vi "solar_msg Q Obtain.vi"(7 "Max Queue Size (-1, unlimited)":i32=-1, 8 "error in (no error)":errorcluster, 9 "Create If Not Found? (T)":bool=TRUE, 11 "Queue Name (unnamed)":string) -> (0 "error out":errorcluster, 1 "Created New?":bool, 3 "Queue":refnum<queue>)   [LabVIEW 2018]
doc: "This obtains a queue reference by name."
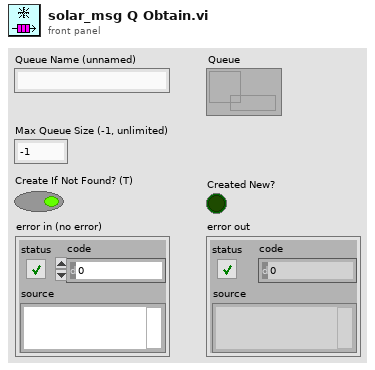
[diagram p1: front panel]
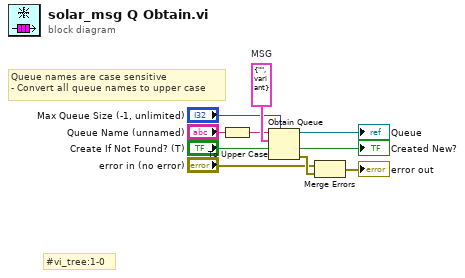
[diagram p0: block diagram]
diagram:
  w10 = cluster{"MSG":string, "DATA":variant} {"MSG"="", "DATA"=variant}  # MSG
  # "#vi_tree:1-0"
  # "Queue names are case sensitive\n- Convert all queue names to upper case"
  n1 = To Upper Case(1:"Queue Name (unnamed)") -> (0:w1:string)
  n2 = Obtain Queue(max queue size (-1, unlimited)="Max Queue Size (-1, unlimited)", name (unnamed)=w1, element data type=w10, create if not found? (T)="Create If Not Found? (T)") -> (queue out=→"Queue":refnum<queue>, created new?=→"Created New?":bool, error out=w5:errorcluster)  [unwired: 1 in]
  n3 = Merge Errors("error in (no error)", w5) -> (→"error out":errorcluster)
